vi "输入数据判定.vi"(5 "semaphore":T1, 6 "Socket":dbl, 7 "主从选择":u16(ring) items=["主板", "从板"], 8 "主板选项":string="项目信息", 9 "进度引用":refnum<vi>, 10 "从板个数":dbl=1.0, 11 "错误代码":u32) -> (3 "读取超时":bool)   [LabVIEW 2013]
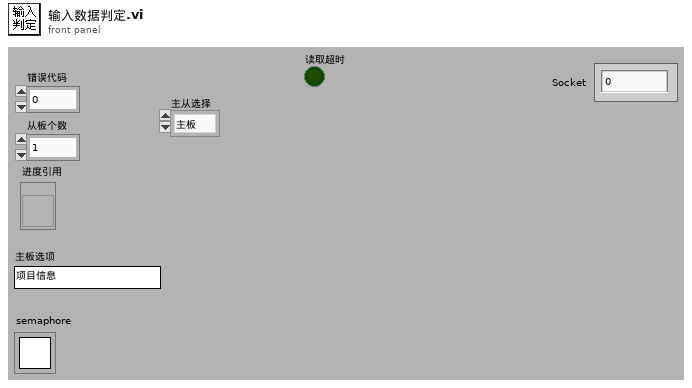
[diagram p1: front panel]
types:
  T1 = typedef "Semaphore RefNum" = refnum<k1>
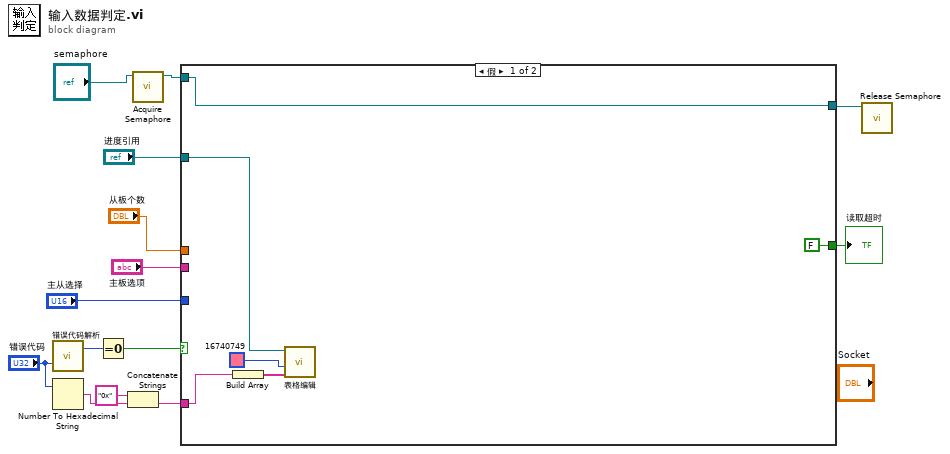
[diagram p0: block diagram]
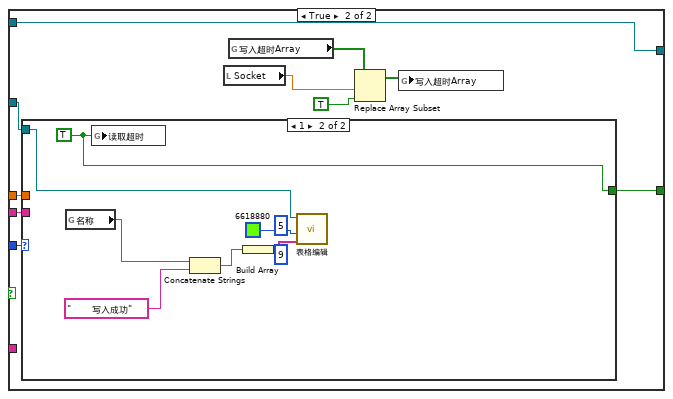
[diagram p2: hidden frame]
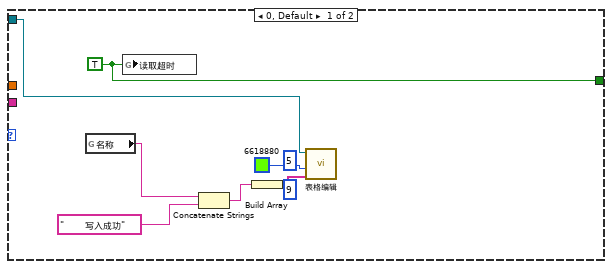
[diagram p3: hidden frame]
diagram:
  n1 = call "错误代码解析.vi"("错误代码"="错误代码") -> ("错误代码"=w10:i32)  [unwired: 2 out]
  n2 = Number To Hexadecimal String(2:"错误代码") -> (0:w8:string)  [unwired: 1 out]
  n3 = Equal To 0?(x=w10) -> (x = 0?=w11:bool)
  n4 = Concatenate Strings("0x" ("字符串"), w8) -> (w7:string)
  n5 = call <vilib>:"Acquire Semaphore.vi"("semaphore"="semaphore") -> ("semaphore out"=w3:T1)  [unwired: 4 in, 2 out]
  n6 = case shown="假" w11 {
    tunnel: "主板选项" -> [_ w30]
    tunnel: "进度引用" -> [w17 w29]
    tunnel: "从板个数" -> [_ w28]
    tunnel: "主从选择" -> [_ w27]
    tunnel: w7 -> [w20 _]
    tunnel: [w16 w22] -> w2
    tunnel: w3 -> [w16 w22]
    tunnel: [FALSE ("读取超时") w21] -> w1
    frame False {
      n7 = Build Array(w20) -> (w19:string[])
      n8 = call "表格编辑.vi"("新元素/子数组"=w19, "活动单元格:单元格背景色"=u32 16740749, "MCListbox引用句柄"=w17) -> ()  [unwired: 9 out]
    }
    frame True {
      n9 = case shown="1" w27 {
        tunnel: w30 -> [_ _]
        tunnel: w29 -> [w33 w40]
        tunnel: w28 -> [_ _]
        tunnel: [w31 w38] -> w21
        frame 0, Default {
          (unwired) u32 9 ("表格总行数")
          (unwired) 5 ("保留行数")
          w31 = TRUE ("读取超时")
          n10 = global read "全局 1.vi" "名称"() -> (w32:string)
          n11 = global write "EV05全局变量1.vi" "读取超时"(w31) -> ()
          n12 = Concatenate Strings(w32, "       写入成功" ("字符串")) -> (w36:string)
          n13 = Build Array(w36) -> (w35:string[])
          n14 = call "表格编辑.vi"("新元素/子数组"=w35, "活动单元格:单元格背景色"=u32 6618880, "MCListbox引用句柄"=w33) -> ()  [unwired: 9 out]
        }
        frame 1 {
          (unwired) u32 9 ("表格总行数")
          (unwired) 5 ("保留行数")
          w38 = TRUE ("读取超时")
          n15 = global read "全局 1.vi" "名称"() -> (w39:string)
          n16 = global write "EV05全局变量1.vi" "读取超时"(w38) -> ()
          n17 = Concatenate Strings(w39, "       写入成功" ("字符串")) -> (w43:string)
          n18 = Build Array(w43) -> (w42:string[])
          n19 = call "表格编辑.vi"("新元素/子数组"=w42, "活动单元格:单元格背景色"=u32 6618880, "MCListbox引用句柄"=w40) -> ()  [unwired: 9 out]
        }
      }
      n20 = local read "Socket"() -> (w24:dbl)
      n21 = global read "EV05全局变量1.vi" "写入超时Array"() -> (w25:bool[])
      n22 = Replace Array Subset(array=w25, new element=TRUE ("写入超时"), index=w24) -> (w26:bool[])
      n23 = global write "EV05全局变量1.vi" "写入超时Array"(w26) -> ()
    }
  }
  "读取超时" <- w1
  n24 = call <vilib>:"Release Semaphore.vi"("semaphore"=w2) -> ()  [unwired: 5 in, 2 out]
